vi "LAUNCH.vi"() -> ()   [LabVIEW 2020]
uses:
  <userlib>/_NEVSTOP/Communicable State Machine(CSM)/Communicable State Machine.lvlib
  <vilib>/Utility/config.llb/NI_LVConfig.lvlib
  <vilib>/Utility/config.llb/Read Key (String).vi
  <vilib>/Utility/config.llb/Write Key (String).vi
  <userlib>/_NEVSTOP/Communicable State Machine(CSM)/_Polymophic/Build No-Reply Asynchronous Message with Arguments.vi
panel:
  out "State History":string
  in  "exit":bool
  in  "login":bool
  in  "register":bool
  in  "password":string
  in  "username":string
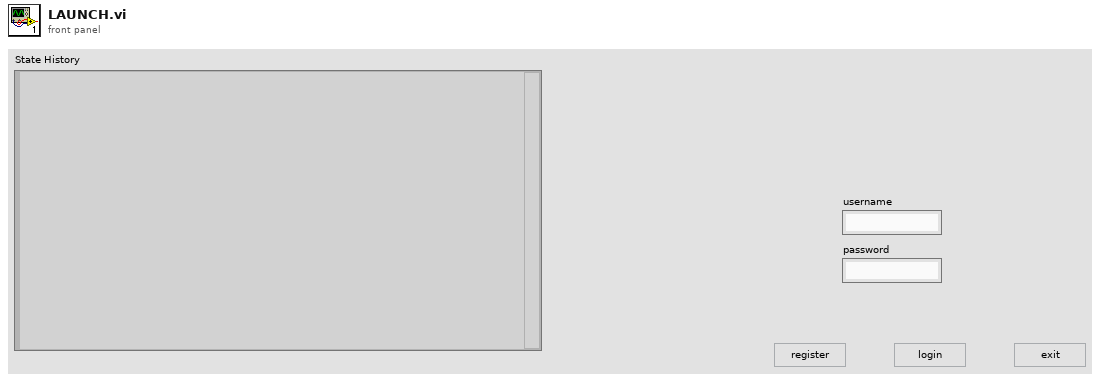
[diagram p1: front panel]
types:
  T1 = enum32{"Invalid", "Standard", "Closed", "Hidden", "Minimized", "Maximized"}
  T2 = enum32{"invalid app kind", "Development System", "Run Time System", "Student Edition", "Embedded LabVIEW", "Evaluation", "Custom"}
  T3 = typedef "Communicable State Machine.lvlib/_CSM_Response Source Message.ctl" = cluster{"‘State":string, "’Arguments":string, "’Error":errorcluster}
  T4 = typedef "NI_LVConfig.lvlib/Config Data RefNum.ctl" = refnum<k1>
  T5 = cluster{"Core":cluster{"Current VI Reference":refnum<vi>, "Close Panel on Exit?":bool}, "Your Boolean data":bool, "username":string}
  T6 = cluster{"Current VI Reference":refnum<vi>, "Close Panel on Exit?":bool}
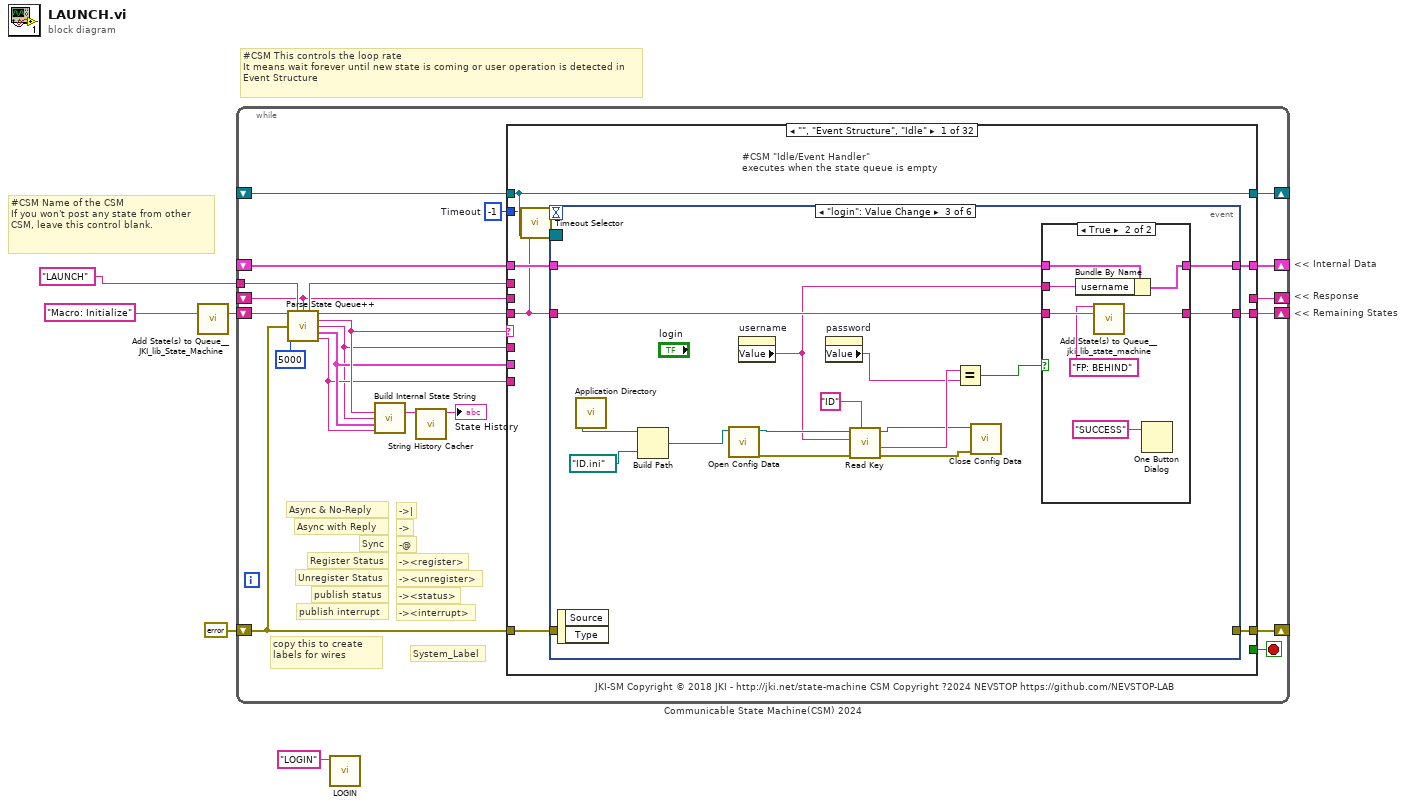
[diagram p0: block diagram]
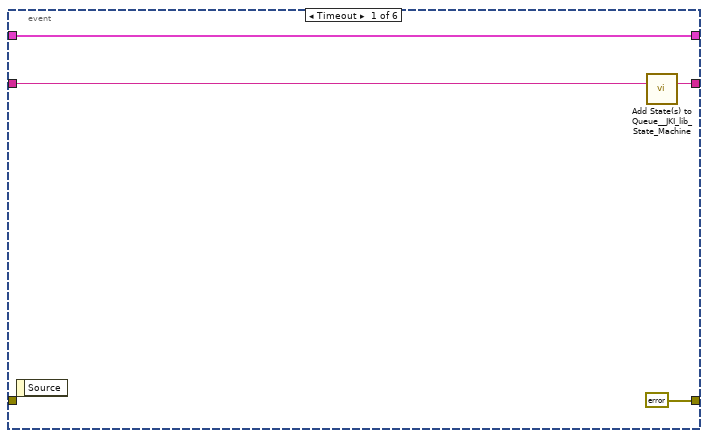
[diagram p2: hidden frame]
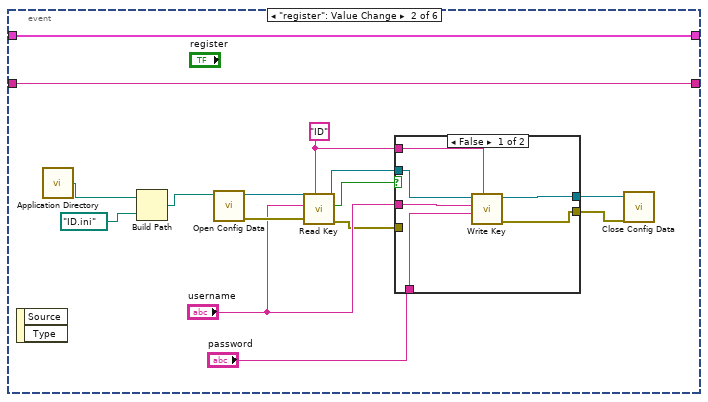
[diagram p3: hidden frame]
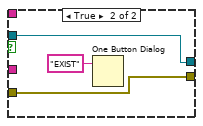
[diagram p4: hidden frame]
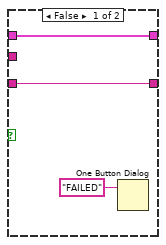
[diagram p5: hidden frame]
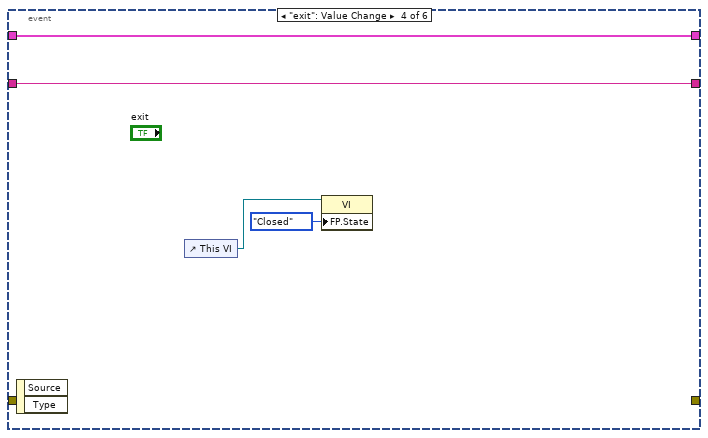
[diagram p6: hidden frame]
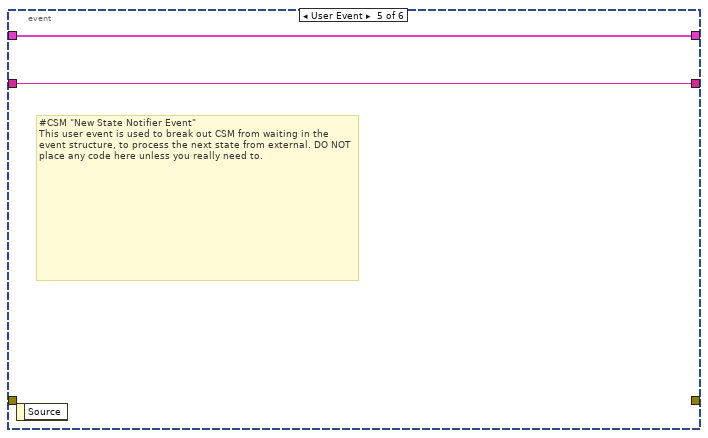
[diagram p7: hidden frame]
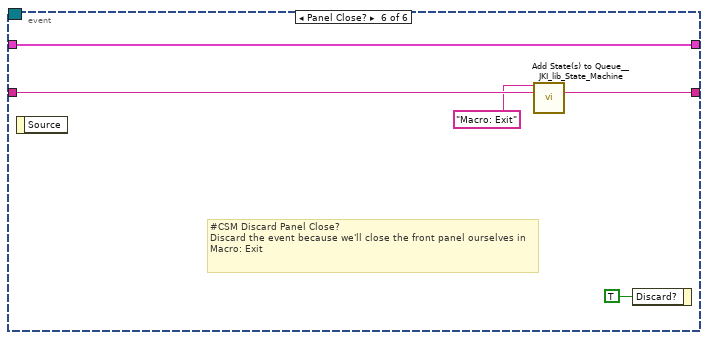
[diagram p8: hidden frame]
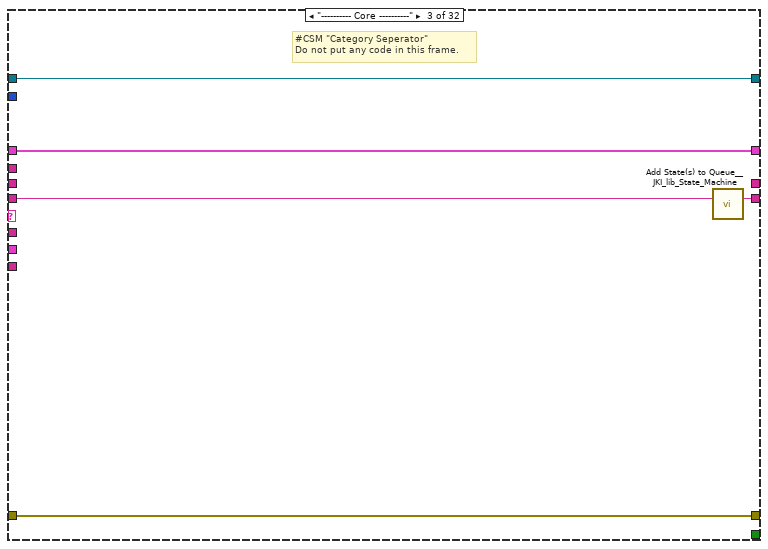
[diagram p10: hidden frame]
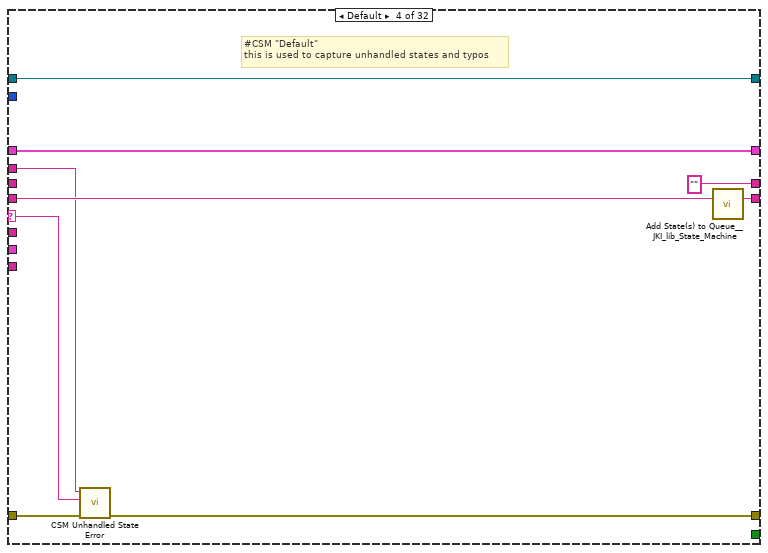
[diagram p11: hidden frame]
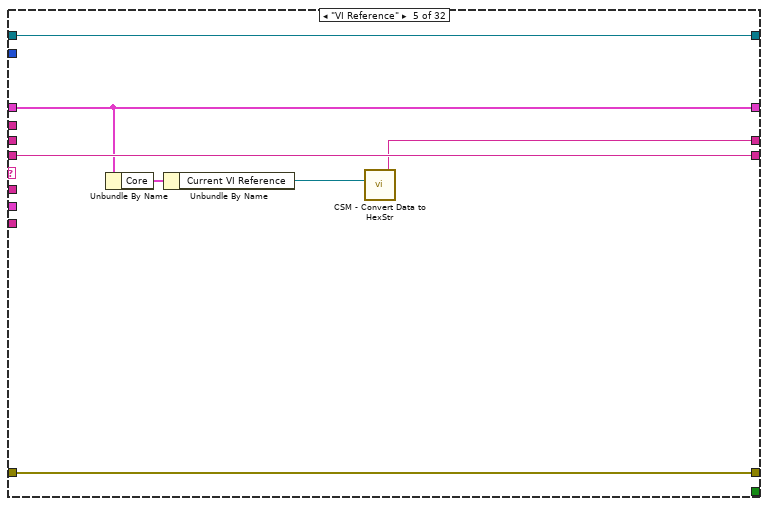
[diagram p12: hidden frame]
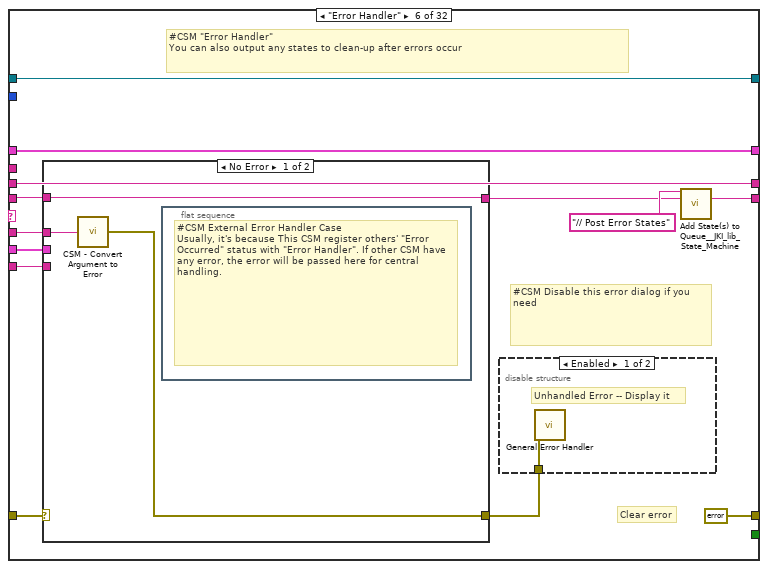
[diagram p13: hidden frame]
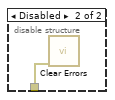
[diagram p14: hidden frame]
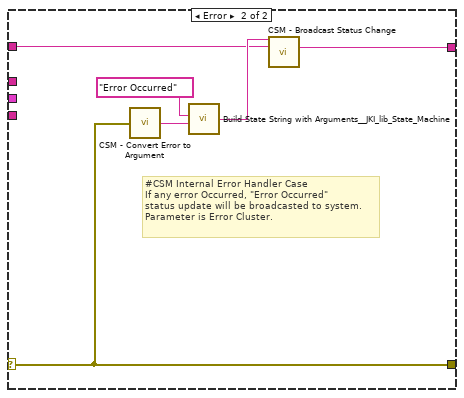
[diagram p15: hidden frame]
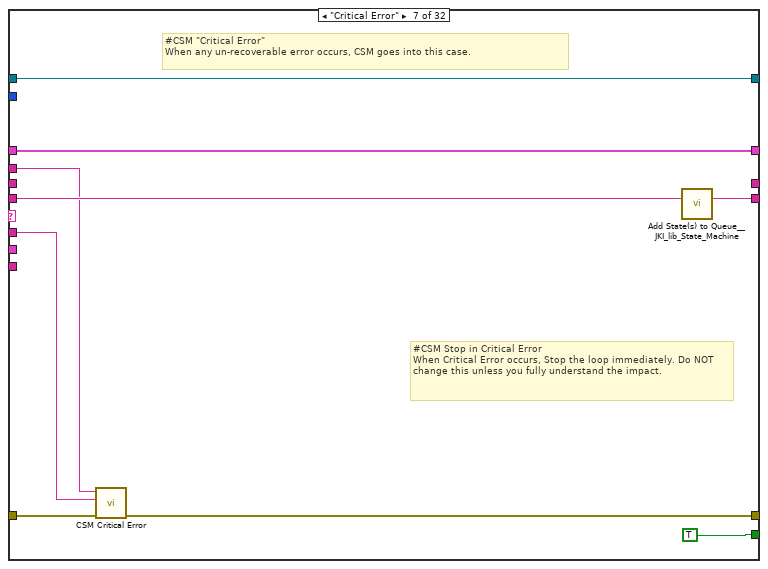
[diagram p16: hidden frame]
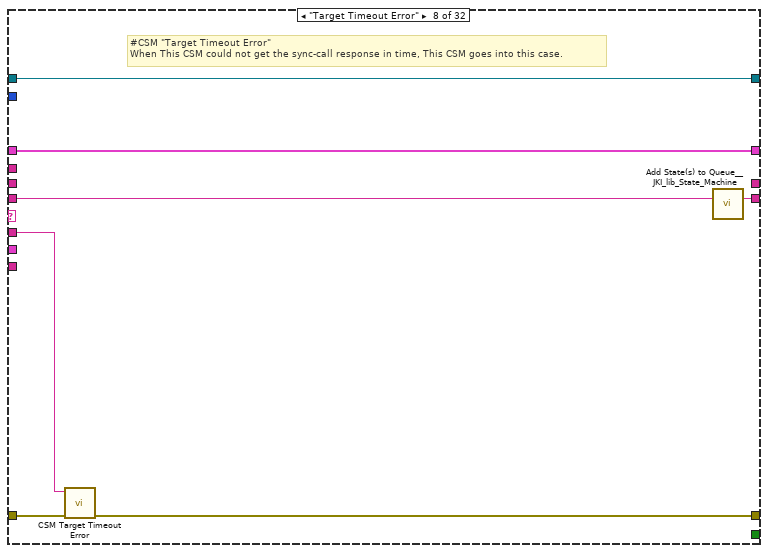
[diagram p17: hidden frame]
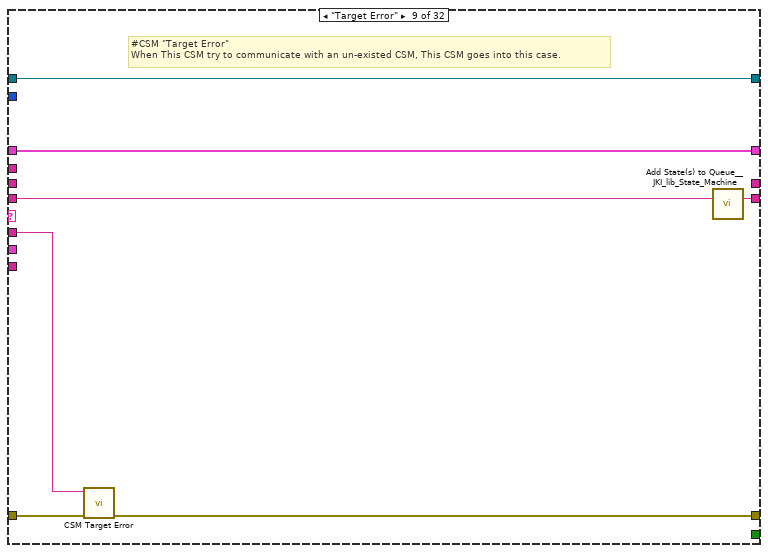
[diagram p18: hidden frame]
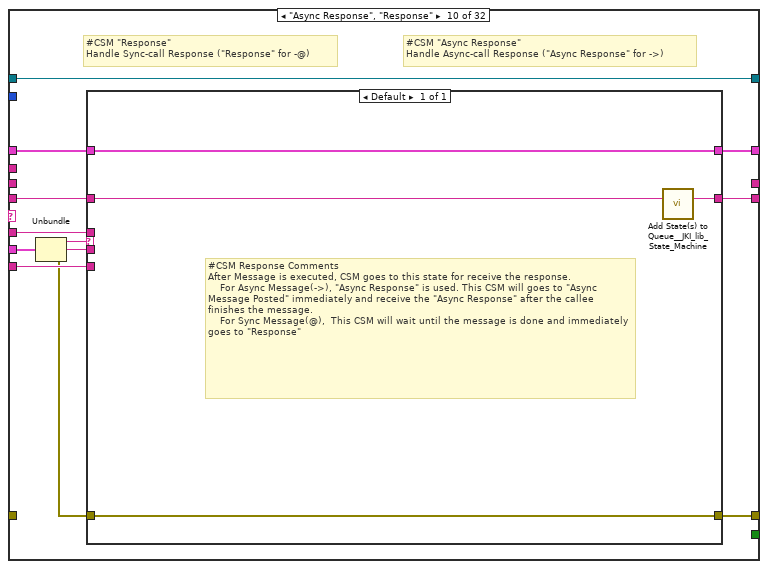
[diagram p19: hidden frame]
diagram:
  # "<< Internal Data"
  # "<< Response"
  # "<< Remaining States"
  # "#CSM Name of the CSM\nIf you won't post any state from other CSM, leave this control blank."
  # "#CSM This controls the loop rate\nIt means wait forever until new state is coming or user operation is detected in Event Structure"
  n1 = call <vilib>:"Add State(s) to Queue__JKI_lib_State_Machine.vi"("State(s) in (\"\")"="Macro: Initialize" ("Init State(\"Macro: Initialize\")")) -> ("States Out"=w4:string)  [unwired: 14 in]
  n2 = while "Communicable State Machine(CSM) 2024" {
    shift-right: [w22] -> _
    shift-left: _ -> [w21]
    shift-right: [w25] -> _
    shift-left: errorcluster {"status"=FALSE, "code"=0, "source"=""} ("error out") -> [w19]
    shift-right: [w24] -> _
    shift-left: w4 -> [w26]
    tunnel: "LAUNCH" ("Name(\"\" to use uuid)") -> [w14]
    shift-right: [w17] -> _
    shift-left: _ -> [w7]
    shift-right: [w16] -> _
    shift-left: _ -> [w15]
    stop <- w23 stop-if-true
    w20 = -1  # Timeout
    # "-><interrupt>"
    # "-><status>"
    # "-><unregister>"
    # "-><register>"
    # "-@"
    # "->"
    # "->|"
    # "publish interrupt"
    # "publish status"
    # "Unregister Status"
    # "Register Status"
    # "Sync"
    # "Async with Reply"
    # "Async & No-Reply"
    # "copy this to create labels for wires"
    # "System_Label"
    # "JKI-SM Copyright © 2018 JKI - http://jki.net/state-machine CSM Copyright ?2024 NEVSTOP https://github.com/NEVSTOP-LAB"
    n3 = call <userlib>:"Parse State Queue++.vi"("State Queue"=w26, "Name(\"\" to use uuid)"=w14, "Response Arguments"=w7, "Error In (no error)"=w19, "Response Timeout(5000ms)"=5000 ("Response Timeout(1000ms)")) -> ("Name Used"=w8:string, "Remaining States"=w27:string, "Current State"=w11:string, "Arguments"=w6:string, ">> Response Source Message >>"=w10:T3, ">> Source CSM >>"=w9:string)  [unwired: 5 in]
    n4 = call <userlib>:"Build Internal State String.vi"("State"=w11, "Arguments (\"\")"=w6, ">> Response Source Message >>"=w10, "Source (\"\")"=w9) -> ("State with Arguments"=w12:string)  [unwired: 11 in]
    n5 = call <userlib>:"String History Cacher.vi"("String"=w12) -> ("String Cache"=→"State History":string)  [unwired: 10 in]
    n6 = case shown="\"\", \"Event Structure\", \"Idle\"" w11 {
      selector: w11 -> [_ _ _ w112 _ _ _ _ _ _ _ _ _ _ _ _ _ _ _ _ _ _ _ _ _ _ _ _ _ _ _ _]
      tunnel: w27 -> [w29 w104 w109 w118 w124 w131 w157 w165 w172 w182 w191 w204 w209 w213 w220 w226 w230 w237 w241 w245 w249 w255 w267 w331 w336 w347 w350 w357 w365 w373 w377 w381]
      tunnel: w6 -> [_ _ _ _ _ w129 w153 w160 w168 w176 _ _ _ _ _ _ _ _ _ _ _ w251 w262 _ _ _ _ _ _ _ _ _]
      tunnel: w21 -> [w35 w103 w106 w116 w123 w137 w158 w163 w170 w180 w190 w198 w207 w211 _ w222 w228 w236 w240 w243 w247 w253 w264 w329 w334 w345 w349 w356 w363 w371 w375 w379]
      tunnel: [w34 _ w107 w110 w125 errorcluster {"status"=FALSE, "code"=0, "source"=""} ("error out") w150 w159 w166 w179 _ _ _ _ _ w223 _ w231 w239 _ _ w252 w265 _ _ _ _ w351 w358 _ _ _] -> w25
      tunnel: w19 -> [w28 _ w107 w111 w125 w135 w151 w161 w167 _ _ _ _ _ _ _ _ _ _ _ _ _ _ _ _ _ _ w352 w359 _ _ _]
      tunnel: [w36 w104 w108 w117 w124 w133 w156 w164 w171 w183 w191 w203 w208 w212 w219 w225 w229 w237 w241 w244 w248 w254 w266 w330 w335 w346 w350 w357 w366 w372 w376 w380] -> w24
      tunnel: [_ _ _ _ _ _ TRUE _ _ _ _ _ TRUE _ _ _ _ _ _ _ _ _ _ _ _ _ _ _ _ _ _ _] -> w23
      tunnel: [w33 w103 w106 w116 w123 w137 w158 w163 w170 w181 w190 w202 w207 w211 w218 w222 w228 w236 w240 w243 w247 w253 w264 w329 w334 w345 w349 w356 w363 w371 w375 w379] -> w22
      tunnel: w20 -> [w31 _ _ _ _ _ _ _ _ _ _ _ _ _ _ _ _ _ _ _ _ _ _ _ _ _ _ _ _ _ _ _]
      tunnel: w9 -> [_ _ _ _ _ w128 _ _ _ w177 _ _ _ _ _ _ _ _ _ _ _ _ _ _ _ _ _ _ _ _ _ _]
      tunnel: w10 -> [_ _ _ _ _ w127 _ _ _ w178 _ _ _ _ _ _ _ _ _ _ _ _ _ _ _ _ _ _ _ _ _ _]
      tunnel: [_ _ _ "" w119 w126 _ _ _ _ _ _ _ _ _ _ _ _ _ _ _ _ _ _ _ _ _ _ _ _ _ _] -> w17
      tunnel: [w32 w102 w105 w114 w122 w136 w154 w162 w169 w184 w189 w192 w205 w210 w214 w221 w227 w235 w238 w242 w246 w250 w261 w328 w332 w338 w348 w355 w369 w370 w374 w378] -> w16
      tunnel: w15 -> [w32 w102 w105 w114 w122 w136 w154 w162 w169 w184 w189 w192 w205 w210 w214 w221 w227 _ w238 w242 w246 w250 w261 w328 w332 w338 w348 w355 w369 w370 w374 w378]
      tunnel: w8 -> [_ _ _ w113 _ _ w152 _ _ _ _ _ _ _ _ _ _ w234 _ _ _ _ _ _ _ _ _ _ _ _ _ _]
      tunnel: w7 -> [_ _ _ _ _ w126 _ _ _ _ _ _ _ _ _ _ _ _ _ _ _ _ _ _ _ _ _ _ _ _ _ _]
      frame "", "Event Structure", "Idle" {
        # "#CSM \"Idle/Event Handler\"\nexecutes when the state queue is empty"
        n7 = call <userlib>:"Timeout Selector.vi"("Remaining States"=w29, "Timeout Expected"=w31) -> ("Timeout"=w30:i32)  [unwired: 5 in]
        n8 = event shown="[2] \"login\": Value Change" {
          selector: w32 -> [_ _ _ _ _ _]
          dyn-events: _ -> [_ _ _ _ _ _]
          timeout: w30 -> [_ _ _ _ _ _]
          tunnel: w29 -> [w40 w55 w68 w94 w95 w101]
          tunnel: [w39 w55 w69 w94 w95 w100] -> w36
          tunnel: w35 -> [w38 w54 w66 w93 w96 w99]
          tunnel: [errorcluster {"status"=FALSE, "code"=0, "source"=""} ("error out") _ _ _ _ _] -> w34
          tunnel: [w38 w54 w67 w93 w96 w99] -> w33
          tunnel: w28 -> [_ _ _ _ _ _]
          event Timeout {
            n9 = event-data() -> ()  [unwired: 1 in, 1 out]
            n10 = call <vilib>:"Add State(s) to Queue__JKI_lib_State_Machine.vi"("State(s) in (\"\")"=w40) -> ("States Out"=w39:string)  [unwired: 14 in]
          }
          event "register": Value Change {
            w45 = "ID" ("section")
            n11 = event-data() -> ()  [unwired: 1 in, 2 out]
            n12 = call <vilib>:"Application Directory.vi"() -> ("Application Directory"=w53:path)
            n13 = Build Path(base path=w53, name or relative path=path "ID.ini") -> (appended path=w51:path)
            n14 = call <vilib>:"Open Config Data.vi"("configuration file path"=w51) -> ("error out"=w49:errorcluster, "refnum"=w50:T4)  [unwired: 8 in, 1 out]
            n15 = call-poly <vilib>:"Read Key.vi"("section"=w45, "error in (no error)"=w49, "key"="username", "refnum"=w50) -> ("error out"=w42:errorcluster, "found?"=w48:bool, "refnum out"=w41:T4)  [unwired: 4 in, 1 out]
            n16 = case shown="False" w48 {
              tunnel: "password" -> [w61 _]
              tunnel: "username" -> [w60 _]
              tunnel: w45 -> [w59 _]
              tunnel: [w58 w63] -> w44
              tunnel: [w57 w62] -> w43
              tunnel: w42 -> [_ w63]
              tunnel: w41 -> [w56 w62]
              frame False {
                n17 = call-poly <vilib>:"Write Key.vi"("section"=w59, "value"=w61, "key"=w60, "refnum"=w56) -> ("error out"=w58:errorcluster, "refnum out"=w57:T4)  [unwired: 5 in, 1 out]
              }
              frame True {
                n18 = One Button Dialog(message="EXIST") -> ()  [unwired: 1 in, 1 out]
              }
            }
            n19 = call <vilib>:"Close Config Data.vi"("error in (no error)"=w44, "refnum"=w43) -> ()  [unwired: 8 in, 2 out]
          }
          event "login": Value Change {
            n20 = event-data() -> ()  [unwired: 1 in, 2 out]
            n21 = call <vilib>:"Application Directory.vi"() -> ("Application Directory"=w80:path)
            n22 = Build Path(base path=w80, name or relative path=path "ID.ini") -> (appended path=w78:path)
            n23 = call <vilib>:"Open Config Data.vi"("configuration file path"=w78) -> ("error out"=w76:errorcluster, "refnum"=w77:T4)  [unwired: 8 in, 1 out]
            n24 = property on="username" class="Str"() -> ("Value"=w65:string)  [unwired: 2 in, 2 out]
            n25 = property on="password" class="Str"() -> ("Value"=w74:string)  [unwired: 2 in, 2 out]
            n26 = call-poly <vilib>:"Read Key.vi"("section"="ID", "error in (no error)"=w76, "key"=w65, "refnum"=w77) -> ("error out"=w73:errorcluster, "value"=w75:string, "refnum out"=w72:T4)  [unwired: 4 in, 1 out]
            n27 = Equal?(x=w75, y=w74) -> (x = y?=w71:bool)
            n28 = call <vilib>:"Close Config Data.vi"("error in (no error)"=w73, "refnum"=w72) -> ()  [unwired: 8 in, 2 out]
            n29 = case shown="True" w71 {
              tunnel: [w82 w89] -> w69
              tunnel: w68 -> [w82 w88]
              tunnel: [w81 w85] -> w67
              tunnel: w66 -> [w81 w86]
              tunnel: w65 -> [_ w84]
              frame False {
                n30 = One Button Dialog(message="FAILED") -> ()  [unwired: 1 in, 1 out]
              }
              frame True {
                n31 = Bundle By Name(cluster=w86, "username"=w84) -> (w85:T5)
                n32 = call <vilib>:"Add State(s) to Queue__jki_lib_state_machine.vi"("State(s) in Front (\"\")"="FP: BEHIND" ("State(s) in Front (\"\")"), "State(s) in (\"\")"=w88) -> ("States Out"=w89:string)  [unwired: 13 in]
                n33 = One Button Dialog(message="SUCCESS") -> ()  [unwired: 1 in, 1 out]
              }
            }
          }
          event "exit": Value Change {
            n34 = event-data() -> ()  [unwired: 1 in, 2 out]
            n35 = control-ref of="This VI"() -> (w92:refnum<vi>)
            n36 = property class="VI"(reference=w92, "FP.State"=T1."Closed" ("Front Panel Window:State")) -> ()  [unwired: 1 in, 2 out]
          }
          event User Event {
            # "#CSM \"New State Notifier Event\"\nThis user event is used to break out CSM from waiting in the event structure, to process the next state from external. DO NOT place any code here unless you really need to."
            n37 = event-data() -> ()  [unwired: 1 in, 1 out]
          }
          event Panel Close? {
            # "#CSM Discard Panel Close?\nDiscard the event because we'll close the front panel ourselves in Macro: Exit"
            n38 = event-data() -> ()  [unwired: 1 in, 1 out]
            n39 = call <vilib>:"Add State(s) to Queue__JKI_lib_State_Machine.vi"("State(s) in Front (\"\")"="Macro: Exit", "State(s) in (\"\")"=w101) -> ("States Out"=w100:string)  [unwired: 13 in]
            n40 = event-data("Discard?"=TRUE) -> ()  [unwired: 1 in, 1 out]
          }
        }
      }
      frame "CSM Documentation" {
        # "#CSM Documentation"
        # "#CSM State Syntax\n\n// Comment line, all text to the right of “//” will be ignored\n// Local Message Example\nDoSth: DoA >> Arguments\n\n// Sync Call Example\nAPI: xxxx >> Arguments -@ TargetModule\n\n// Async Call Example\nAPI: xxxx >> Arguments -> TargetModule\n\n// Async Call without Reply Example\nAPI: xxxx >> Arguments ->| TargetModule\n\n// Broadcast normal status:\nStatus >> StatusArguments  -><status>\n\n// Broadcast Interrupt status:\nInterrupt >> StatusArguments  -><interrupt>\n\n// Register Source Module's status to Handler Module\nStatus@Source Module >> Handler Module@Handler Module -><register>\n\n// Unegister Source Module's status\nStatus@Source Module >> Handler Module -><unregister>"
        # "#CSM README FIRST\n\nCommunicable State Machine(CSM) is a LabVIEW application framework that builds upon JKI State Machine(JKISM). It follows the pattern of JKISM and extends the keywords to describe message communication between modules, including concepts such as Sync-Message, Async-Message, Subscription/Unsubscription of status - essential elements for creating reusable code modules. For more information, please visit the CSM wiki: https://nevstop-lab.github.io/CSM-Wiki/\n\nFor instructions on JKI State Machine, visit: \n    http://jki.net/state-machine/\nFor information about CSM, visit: \n    https://github.com/NEVSTOP-LAB"
        # "#CSM \"Documentation\"\nCase for holding CSM Documenation"
      }
      frame "---------- Core ----------" {
        # "#CSM \"Category Seperator\"\nDo not put any code in this frame."
        n41 = call <vilib>:"Add State(s) to Queue__JKI_lib_State_Machine.vi"("State(s) in (\"\")"=w109) -> ("States Out"=w108:string)  [unwired: 14 in]
      }
      frame Default {
        # "#CSM \"Default\"\nthis is used to capture unhandled states and typos"
        n42 = call <userlib>:"CSM Unhandled State Error.vi"("error in (no error)"=w111, "Current State"=w112, "CSM Name"=w113) -> ("error out"=w110:errorcluster)  [unwired: 8 in]
        n43 = call <vilib>:"Add State(s) to Queue__JKI_lib_State_Machine.vi"("State(s) in (\"\")"=w118) -> ("States Out"=w117:string)  [unwired: 14 in]
      }
      frame "VI Reference" {
        n44 = Unbundle By Name(w123) -> ("Core"=w121:T6)
        n45 = Unbundle By Name(w121) -> ("Current VI Reference"=w120:refnum<vi>)
        n46 = call <userlib>:"CSM - Convert Data to HexStr.vi"("Variant"=w120) -> ("HEX String (0-9,A-F)"=w119:string)  [unwired: 8 in]
      }
      frame "Error Handler" {
        # "#CSM Disable this error dialog if you need"
        # "#CSM \"Error Handler\"\nYou can also output any states to clean-up after errors occur"
        # "Clear error"
        n47 = case shown="No Error" w135 {
          selector: w135 -> [_ w144]
          tunnel: [w142 w146] -> w132
          tunnel: w131 -> [w142 w145]
          tunnel: [w141 w144] -> w130
          tunnel: w129 -> [w143 _]
          tunnel: w128 -> [_ _]
          tunnel: w127 -> [_ _]
          frame No Error {
            n48 = call <userlib>:"CSM - Convert Argument to Error.vi"("Argument"=w143) -> ("error"=w141:errorcluster)  [unwired: 4 in]
            n49 = flat-sequence {
              frame #0 {
                # "#CSM External Error Handler Case\nUsually, it's because This CSM register others' \"Error Occurred\" status with \"Error Handler\". If other CSM have any error, the error will be passed here for central handling."
              }
            }
          }
          frame Error {
            # "#CSM Internal Error Handler Case \nIf any error Occurred, \"Error Occurred\" \nstatus update will be broadcasted to system.\nParameter is Error Cluster."
            n50 = call <userlib>:"CSM - Convert Error to Argument.vi"("error in (no error)"=w144) -> ("Arguments"=w148:string)  [unwired: 4 in]
            n51 = call <vilib>:"Build State String with Arguments__JKI_lib_State_Machine.vi"("Arguments (\"\")"=w148, "State"="Error Occurred" ("Status with Arguments")) -> ("State with Arguments"=w147:string)  [unwired: 4 in]
            n52 = call <userlib>:"CSM - Broadcast Status Change.vi"("Status with Arguments"=w147, "State Queue"=w145) -> ("Remaining States"=w146:string)  [unwired: 13 in]
          }
        }
        n53 = disable-structure shown="Enabled" {
          disable-tunnel: w130 -> [w139 w140]
          frame Enabled {
            # "Unhandled Error -- Display it"
            n54 = call <vilib>:"General Error Handler.vi"("error in (no error)"=w139) -> ()  [unwired: 10 in, 5 out]
          }
          frame Disabled {
            n55 = call <vilib>:"Clear Errors.vi"("error in (no error)"=w140) -> ()  [unwired: 5 in, 2 out]
          }
        }
        n56 = call <vilib>:"Add State(s) to Queue__JKI_lib_State_Machine.vi"("State(s) in Front (\"\")"="// Post Error States", "State(s) in (\"\")"=w132) -> ("States Out"=w133:string)  [unwired: 13 in]
      }
      frame "Critical Error" {
        # "#CSM \"Critical Error\"\nWhen any un-recoverable error occurs, CSM goes into this case."
        # "#CSM Stop in Critical Error\nWhen Critical Error occurs, Stop the loop immediately. Do NOT change this unless you fully understand the impact."
        n57 = call <userlib>:"CSM Critical Error.vi"("error in (no error)"=w151, "Arugments(as Reason)"=w153, "CSM Name"=w152) -> ("error out"=w150:errorcluster)  [unwired: 8 in]
        n58 = call <vilib>:"Add State(s) to Queue__JKI_lib_State_Machine.vi"("State(s) in (\"\")"=w157) -> ("States Out"=w156:string)  [unwired: 14 in]
      }
      frame "Target Timeout Error" {
        # "#CSM \"Target Timeout Error\"\nWhen This CSM could not get the sync-call response in time, This CSM goes into this case."
        n59 = call <userlib>:"CSM Target Timeout Error.vi"("error in (no error)"=w161, "Arguments(as CSM Name)"=w160) -> ("error out"=w159:errorcluster)  [unwired: 9 in]
        n60 = call <vilib>:"Add State(s) to Queue__JKI_lib_State_Machine.vi"("State(s) in (\"\")"=w165) -> ("States Out"=w164:string)  [unwired: 14 in]
      }
      frame "Target Error" {
        # "#CSM \"Target Error\"\nWhen This CSM try to communicate with an un-existed CSM, This CSM goes into this case."
        n61 = call <userlib>:"CSM Target Error.vi"("error in (no error)"=w167, "Arguments(as CSM Name)"=w168) -> ("error out"=w166:errorcluster)  [unwired: 9 in]
        n62 = call <vilib>:"Add State(s) to Queue__JKI_lib_State_Machine.vi"("State(s) in (\"\")"=w172) -> ("States Out"=w171:string)  [unwired: 14 in]
      }
      frame "Async Response", "Response" {
        # "#CSM \"Async Response\"\nHandle Async-call Response (\"Async Response\" for ->)"
        # "#CSM \"Response\"\nHandle Sync-call Response (\"Response\" for -@)"
        n63 = Unbundle(w178) -> ("‘State"=w175:string, "’Arguments"=w174:string, "’Error"=w173:errorcluster)
        n64 = case shown="Default" w175 {
          tunnel: [w185] -> w183
          tunnel: w182 -> [w186]
          tunnel: [w188] -> w181
          tunnel: w180 -> [w188]
          tunnel: [w187] -> w179
          tunnel: w173 -> [w187]
          tunnel: w177 -> [_]
          tunnel: w176 -> [_]
          tunnel: w174 -> [_]
          frame Default {
            # "#CSM Response Comments\nAfter Message is executed, CSM goes to this state for receive the response.\n    For Async Message(->), \"Async Response\" is used. This CSM will goes to \"Async Message Posted\" immediately and receive the \"Async Response\" after the callee finishes the message.\n    For Sync Message(@),  This CSM will wait until the message is done and immediately goes to \"Response\""
            n65 = call <vilib>:"Add State(s) to Queue__JKI_lib_State_Machine.vi"("State(s) in (\"\")"=w186) -> ("States Out"=w185:string)  [unwired: 14 in]
          }
        }
      }
      frame "Async Message Posted" {
        # "#CSM \"Async Message Posted\"\nAfter Async Message is posted (-> or ->| ), CSM goes to this state for post-action.\nYou can use Argument - State to tell which Async Message is called."
      }
      frame "Initialize Core Data" {
        # "#CSM \"Initialize Core Data\"\nThis is used to determine panel behavior on exit"
        # "originally closed?"
        # "exe?"
        # "If panel starts closed or is an EXE, then close it when we exit"
        n66 = property class="VI"() -> ("FP.State"=w195:T1)  [unwired: 2 in, 2 out]
        n67 = property class="App"() -> ("App.Kind"=w201:T2)  [unwired: 2 in, 2 out]
        n68 = control-ref of="Current VI Reference"() -> (w196:refnum<vi>)
        n69 = Equal?(x=w195, y=T1."Closed" ("Front Panel Window:State")) -> (x = y?=w193:bool)
        n70 = Equal?(x=w201, y=T2."Run Time System" ("Application:Kind")) -> (x = y?=w199:bool)
        n71 = Or(x=w193, y=w199) -> (x .or. y?=w197:bool)
        n72 = Bundle By Name(cluster=w198, "Core.Current VI Reference"=w196, "Core.Close Panel on Exit?"=w197) -> (w202:T5)
        n73 = call <vilib>:"Add State(s) to Queue__JKI_lib_State_Machine.vi"("State(s) in (\"\")"=w204) -> ("States Out"=w203:string)  [unwired: 14 in]
      }
      frame "Exit" {
        # "#CSM \"Exit\"\nCase for exiting the loop. No errors that occur here will be handled."
        n74 = call <vilib>:"Add State(s) to Queue__JKI_lib_State_Machine.vi"("State(s) in (\"\")"=w209) -> ("States Out"=w208:string)  [unwired: 14 in]
      }
      frame "---------- Data ----------" {
        # "#CSM \"Category Seperator\"\nDo not put any code in this frame."
        n75 = call <vilib>:"Add State(s) to Queue__JKI_lib_State_Machine.vi"("State(s) in (\"\")"=w213) -> ("States Out"=w212:string)  [unwired: 14 in]
      }
      frame "Data: Initialize" {
        w215 = T6 {"Current VI Reference"=refnum, "Close Panel on Exit?"=FALSE}  # Core
        w217 = TRUE  # Your Boolean data
        w216 = ""  # username
        # "#CSM  do not delete - used by framework"
        # "#CSM Expand Bundle to add new data elements to shift register data."
        # "#CSM Add new data here."
        # "#CSM Data names and types of shift register data are defined by this bundle."
        # "#CSM \"Data: Initialize\"\nInitialize the shift-register data, here.\n(data names are defined by what you wire into the bundle function)"
        n76 = Bundle("Core"=w215, "Your Boolean data"=w217, "username"=w216) -> (w218:T5)  [unwired: 1 in]
        n77 = call <vilib>:"Add State(s) to Queue__JKI_lib_State_Machine.vi"("State(s) in (\"\")"=w220) -> ("States Out"=w219:string)  [unwired: 14 in]
      }
      frame "Data: Cleanup" {
        # "#CSM \"Data: Cleanup\"\nCleanup any data and references, here.\n(this is called automatically, by the Macro: Exit)"
        n78 = Unbundle By Name(w222) -> ("Core.Current VI Reference"=w224:refnum<vi>)
        n79 = Close Reference(reference=w224) -> (error out=w223:errorcluster)  [unwired: 1 in]
        n80 = call <vilib>:"Add State(s) to Queue__JKI_lib_State_Machine.vi"("State(s) in (\"\")"=w226) -> ("States Out"=w225:string)  [unwired: 14 in]
      }
      frame "---------- Events ----------" {
        # "#CSM \"Category Seperator\"\nDo not put any code in this frame."
        n81 = call <vilib>:"Add State(s) to Queue__JKI_lib_State_Machine.vi"("State(s) in (\"\")"=w230) -> ("States Out"=w229:string)  [unwired: 14 in]
      }
      frame "Events: Register" {
        # "#CSM \"Events: Register\"\nRegister user event. New Message Event is registered to break CSM waiting in event structure by default."
        # "#CSM Register New Message Event\nRegister message event to break Waiting in Event structure."
        n82 = call <userlib>:"CSM - Get New State Notifier Event.vi"("Name(\"\" to use uuid) in"=w234) -> ("Error out"=w232:errorcluster, "New State Notifier Event"=w233:refnum<user-event>)  [unwired: 9 in]
        n83 = register-events(error in=w232, w233) -> (reference out=w235:refnum<event-registration>, error out=w231:errorcluster)  [unwired: 1 in]
      }
      frame "Events: Unregister" {
        # "#CSM \"Events: Unregister\"\nUnregister user event."
        n84 = Unregister For Events(event registration refnum=w238) -> (error out=w239:errorcluster)  [unwired: 1 in]
      }
      frame "---------- UI ----------" {
        # "#CSM \"Category Seperator\"\nDo not put any code in this frame."
        n85 = call <vilib>:"Add State(s) to Queue__JKI_lib_State_Machine.vi"("State(s) in (\"\")"=w245) -> ("States Out"=w244:string)  [unwired: 14 in]
      }
      frame "UI: Initialize" {
        # "#CSM \"UI: Initialize\"\nInitialize the User Interface, here.\n(this is called automatically, by the Macro: Init)"
        n86 = call <vilib>:"Add State(s) to Queue__JKI_lib_State_Machine.vi"("State(s) in (\"\")"=w249) -> ("States Out"=w248:string)  [unwired: 14 in]
      }
      frame "UI: Cursor Set" {
        # "Argument"
        # "#CSM \"UI: Cursor Set\"\nSet and Unset Cursor Busy.\n(Usage: \"UI: Cursor Set >> Busy|Idle\")"
        n87 = disable-structure shown="Default" {
          disable-tunnel: [w257 w260] -> w252
          disable-tunnel: w251 -> [w256 _]
          frame condition #0 (active) {
            n88 = case shown="\"Idle\", Default" w256 {
              tunnel: [w258 w259] -> w257
              frame "Idle", Default {
                n89 = call <vilib>:"Unset Busy.vi"() -> ("error out"=w258:errorcluster)  [unwired: 11 in]
              }
              frame "Busy" {
                n90 = call <vilib>:"Set Busy.vi"() -> ("error out"=w259:errorcluster)  [unwired: 10 in, 1 out]
              }
            }
          }
          frame condition #1 {
          }
        }
        n91 = call <vilib>:"Add State(s) to Queue__JKI_lib_State_Machine.vi"("State(s) in (\"\")"=w255) -> ("States Out"=w254:string)  [unwired: 14 in]
      }
      frame "UI: Front Panel State" {
        # "Argument"
        # "#CSM \"UI: Front Panel State\"\nSet Front Panel Open or Closed\n(Usage: \"UI: Front Panel State >> Open|Close\")"
        n92 = Unbundle By Name(w264) -> ("Core.Current VI Reference"=w263:refnum<vi>)
        n93 = case shown="\"Minimize\", \"Minimized\"" w262 {
          tunnel: [w274 w287 w298 w310 w322] -> w265
          tunnel: w263 -> [w273 w285 w297 w309 w321]
          frame "Open", "Standard", Default {
            w268 = T1."Standard" ("State")
            n94 = property class="VI"(reference=w273) -> (reference out=w271:refnum<vi>, error out=w272:errorcluster, "FP.State"=w270:T1)  [unwired: 1 in]
            n95 = Not Equal?(x=w270, y=w268) -> (x != y?=w269:bool)
            n96 = case shown="True" w269 {
              tunnel: [w278 w280] -> w274
              tunnel: w272 -> [w277 w280]
              tunnel: w271 -> [w276 _]
              tunnel: w268 -> [w275 _]
              frame True {
                n97 = invoke class="VI" method="FP.Open"(reference=w276, error in=w277, "Activate"=TRUE, "State"=w275) -> (error out=w278:errorcluster)  [unwired: 1 in, 4 out]
              }
              frame False {
              }
            }
          }
          frame "Close", "Closed" {
            n98 = property class="VI"(reference=w285) -> (reference out=w284:refnum<vi>, error out=w286:errorcluster, "FP.State"=w282:T1)  [unwired: 1 in]
            n99 = Not Equal?(x=w282, y=T1."Closed" ("Front Panel Window:State")) -> (x != y?=w281:bool)
            n100 = case shown="True" w281 {
              tunnel: [w288 w291] -> w287
              tunnel: w286 -> [w288 w290]
              tunnel: w284 -> [_ w289]
              frame False {
              }
              frame True {
                n101 = invoke class="VI" method="FP.Close"(reference=w289, error in=w290) -> (error out=w291:errorcluster)  [unwired: 1 in, 2 out]
              }
            }
          }
          frame "Hidden", "Hide" {
            w292 = T1."Hidden" ("State")
            n102 = property class="VI"(reference=w297) -> (reference out=w295:refnum<vi>, error out=w296:errorcluster, "FP.State"=w294:T1)  [unwired: 1 in]
            n103 = Not Equal?(x=w294, y=w292) -> (x != y?=w293:bool)
            n104 = case shown="True" w293 {
              tunnel: [w302 w303] -> w298
              tunnel: w296 -> [w301 w303]
              tunnel: w295 -> [w300 _]
              tunnel: w292 -> [w299 _]
              frame True {
                n105 = invoke class="VI" method="FP.Open"(reference=w300, error in=w301, "State"=w299) -> (error out=w302:errorcluster)  [unwired: 2 in, 4 out]
              }
              frame False {
              }
            }
          }
          frame "Minimize", "Minimized" {
            w304 = T1."Minimized" ("State")
            n106 = property class="VI"(reference=w309) -> (reference out=w307:refnum<vi>, error out=w308:errorcluster, "FP.State"=w306:T1)  [unwired: 1 in]
            n107 = Not Equal?(x=w306, y=w304) -> (x != y?=w305:bool)
            n108 = case shown="True" w305 {
              tunnel: [w314 w315] -> w310
              tunnel: w308 -> [w313 w315]
              tunnel: w307 -> [w312 _]
              tunnel: w304 -> [w311 _]
              frame True {
                n109 = invoke class="VI" method="FP.Open"(reference=w312, error in=w313, "State"=w311) -> (error out=w314:errorcluster)  [unwired: 2 in, 4 out]
              }
              frame False {
              }
            }
          }
          frame "Maximize", "Maximized" {
            w316 = T1."Maximized" ("State")
            n110 = property class="VI"(reference=w321) -> (reference out=w319:refnum<vi>, error out=w320:errorcluster, "FP.State"=w318:T1)  [unwired: 1 in]
            n111 = Not Equal?(x=w318, y=w316) -> (x != y?=w317:bool)
            n112 = case shown="True" w317 {
              tunnel: [w326 w327] -> w322
              tunnel: w320 -> [w325 w327]
              tunnel: w319 -> [w324 _]
              tunnel: w316 -> [w323 _]
              frame True {
                n113 = invoke class="VI" method="FP.Open"(reference=w324, error in=w325, "State"=w323) -> (error out=w326:errorcluster)  [unwired: 2 in, 4 out]
              }
              frame False {
              }
            }
          }
        }
        n114 = call <vilib>:"Add State(s) to Queue__JKI_lib_State_Machine.vi"("State(s) in (\"\")"=w267) -> ("States Out"=w266:string)  [unwired: 14 in]
      }
      frame "---------- Macro ----------" {
        # "#CSM \"Category Seperator\"\nDo not put any code in this frame."
        n115 = call <vilib>:"Add State(s) to Queue__JKI_lib_State_Machine.vi"("State(s) in (\"\")"=w331) -> ("States Out"=w330:string)  [unwired: 14 in]
      }
      frame "Macro: Initialize" {
        w333 = "Data: Initialize\nInitialize Core Data\nEvents: Register\nUI: Initialize\nUI: Front Panel State >> Open"  # Data: Initialize Initialize Core Data Events: Register UI: Initialize UI: Front Panel State >> Open
        # "#CSM \"Macro: Initialize\"\nInitialization Macro (This is called once, when the VI starts)"
        n116 = call <vilib>:"Add State(s) to Queue__JKI_lib_State_Machine.vi"("State(s) in Front (\"\")"=w333, "State(s) in (\"\")"=w336) -> ("States Out"=w335:string)  [unwired: 13 in]
      }
      frame "Macro: Exit" {
        # "#CSM \"Macro: Exit\"\nExit Macro (This is called once, when the VI exits)"
        n117 = Unbundle By Name(w345) -> ("Core.Close Panel on Exit?"=w344:bool)
        n118 = Select(t="UI: Front Panel State >> Close", s=w344, f="") -> (s? t:f=w341:string)
        n119 = call <vilib>:"Add State(s) to Queue__JKI_lib_State_Machine.vi"("State(s) in Front (\"\")"="//Exit Sub-Modules ", "State(s) in (\"\")"=w341, "State(s) at Back (\"\")"="Data: Cleanup\nEvents: Unregister\nExit") -> ("States Out"=w339:string)  [unwired: 12 in]
        n120 = call <vilib>:"Add State(s) to Queue__JKI_lib_State_Machine.vi"("State(s) in Front (\"\")"=w339, "State(s) in (\"\")"=w347) -> ("States Out"=w346:string)  [unwired: 13 in]
      }
      frame "---------- FP ----------" {
        # "#CSM \"Category Seperator\"\nDo not put any code in this frame."
      }
      frame "FP: FRONT" {
        # "#CSM API Example\nCopy/Rename this case for your own API"
        n121 = control-ref of="This VI"() -> (w354:refnum<vi>)
        n122 = property class="VI"(reference=w354, error in=w352, "FP.State"=T1."Standard" ("Front Panel Window:State")) -> (error out=w351:errorcluster)  [unwired: 1 out]
      }
      frame "FP: BEHIND" {
        # "#CSM API Example\nCopy/Rename this case for your own API"
        n123 = Unbundle By Name(w363) -> ("username"=w362:string)
        n124 = control-ref of="This VI"() -> (w361:refnum<vi>)
        n125 = property class="VI"(reference=w361, error in=w359, "FP.State"=T1."Hidden" ("Front Panel Window:State")) -> (error out=w358:errorcluster)  [unwired: 1 out]
        n126 = call-poly <userlib>:"Build Message with Arguments++.vi"("State with Arguments"="FP: FRONT", "Arguments (\"\")"=w362, "Target Module (\"\")"="LOGIN" ("Target Module (\"\")")) -> ("State with Arguments out"=w364:string)  [unwired: 12 in]
        n127 = call <vilib>:"Add State(s) to Queue__jki_lib_state_machine.vi"("State(s) in Front (\"\")"=w364, "State(s) in (\"\")"=w365) -> ("States Out"=w366:string)  [unwired: 13 in]
      }
      frame "---------- Action ----------" {
        # "#CSM \"Category Seperator\"\nDo not put any code in this frame."
        n128 = call <vilib>:"Add State(s) to Queue__JKI_lib_State_Machine.vi"("State(s) in (\"\")"=w373) -> ("States Out"=w372:string)  [unwired: 14 in]
      }
      frame "Action: action1" {
        # "#CSM \"Internal State\"\nThis category is used for holding internal states"
        n129 = call <vilib>:"Add State(s) to Queue__JKI_lib_State_Machine.vi"("State(s) in (\"\")"=w377) -> ("States Out"=w376:string)  [unwired: 14 in]
      }
      frame "Action: action2" {
        # "#CSM \"Internal State\"\nThis category is used for holding internal states"
        n130 = call <vilib>:"Add State(s) to Queue__JKI_lib_State_Machine.vi"("State(s) in (\"\")"=w381) -> ("States Out"=w380:string)  [unwired: 14 in]
      }
    }
  }
  n131 = call "LOGIN.vi"("Name(\"\" to use uuid)"="LOGIN" ("Name(\"\" to use uuid)")) -> ()  [unwired: 11 in]
